vi "Caculates Radius.vi"() -> ()   [LabVIEW 2024]
panel:
  in  "y":i32
  out "Factorial":dbl
  in  "Slide":dbl(slide) scale=0.0..100.0
  out "Temp":dbl
  in  "Increment":dbl
  out "Thermometer":dbl(slide) scale=0.0..100.0
  out "Radius":dbl
  out "Area":dbl
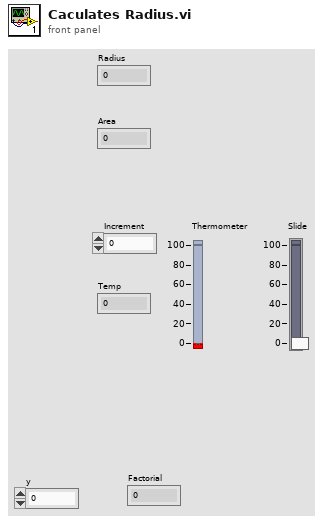
[diagram p1: front panel]
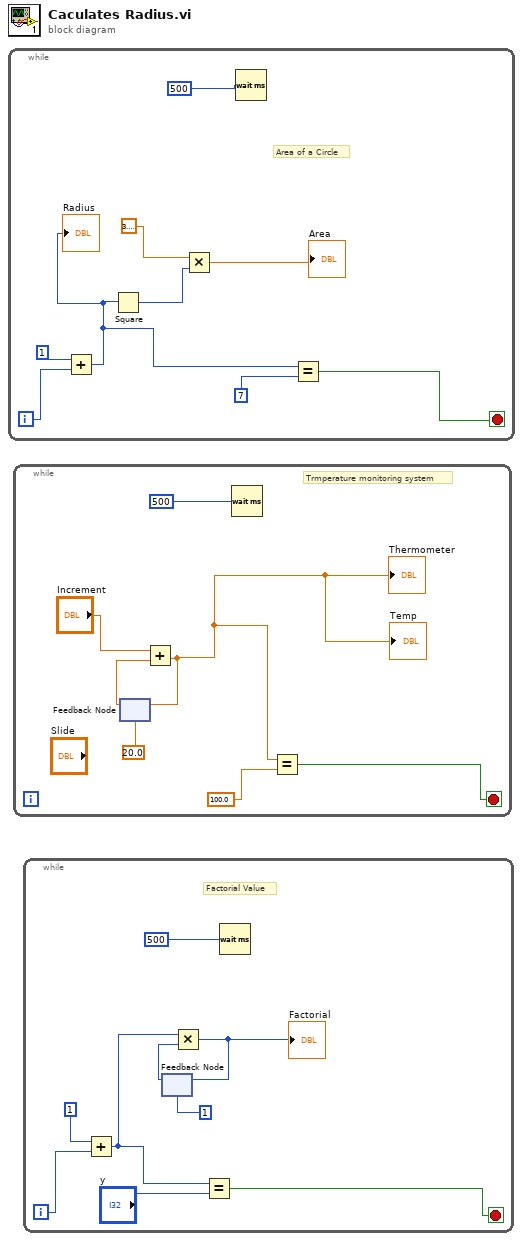
[diagram p0: block diagram]
diagram:
  n1 = while {
    i -> [w9]
    stop <- w3 stop-if-true
    # "Area of a Circle"
    n2 = Add(x=1, y=w9) -> (x+y=w1:i32)
    "Radius" <- w1
    n3 = Square(x=w1) -> (x^2=w7:i32)
    n4 = Multiply(x=3.141592653589793, y=w7) -> (x*y=→"Area":dbl)
    n5 = Wait (ms)(milliseconds to wait=u32 500) -> ()  [unwired: 1 out]
    n6 = Equal?(x=w1, y=7) -> (x = y?=w3:bool)
  }
  n7 = while {
    stop <- w12 stop-if-true
    # "Trmperature monitoring system"
    n8 = feedback #1(20.0) -> (w14:dbl)
    n9 = Add(x="Increment", y=w14) -> (x+y=w11:dbl)
    "Thermometer" <- w11
    "Temp" <- w11
    n10 = feedback-in #1(w11) -> ()
    n11 = Wait (ms)(milliseconds to wait=u32 500) -> ()  [unwired: 1 out]
    n12 = Equal?(x=w11, y=100.0) -> (x = y?=w12:bool)
  }
  n13 = while {
    i -> [w24]
    stop <- w18 stop-if-true
    # "Factorial Value"
    n14 = Add(x=1, y=w24) -> (x+y=w20:i32)
    n15 = feedback #2(1) -> (w25:i32)
    n16 = Multiply(x=w20, y=w25) -> (x*y=w21:i32)
    "Factorial" <- w21
    n17 = feedback-in #2(w21) -> ()
    n18 = Equal?(x=w20, y="y") -> (x = y?=w18:bool)
    n19 = Wait (ms)(milliseconds to wait=u32 500) -> ()  [unwired: 1 out]
  }
